vi "PDP Get Message.vi"(0 "Timeout ms (-1)":i32=-1) -> (1 "PDP Message Type":T1(ring), 2 "Text":string)   [LabVIEW 2009]
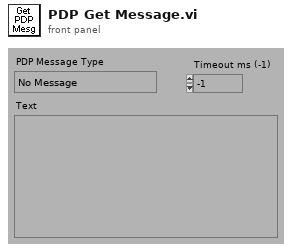
[diagram p1: front panel]
types:
  T1 = enum16{"No Message", "Bad Message", "RFFreq=", "RFMod=", "RFPower=", "QMeterName=", "YaleGain=", "ScanSweeps=", "ScanSteps=", "ScanFreq=", "Material=", "Baseline=", "CalConst=", "MonitorDelay=", "Channel=", "Channels=", "QCAPause", "QCATakeData", "QCANMRTune", "QCAMonitor", "Timer=", "LeadCurrent=", "LeadVoltage=", "MagCurrent=", "MagField=", "MagStatus=", "Setpoint=", "Setrate=", "HeaterDelay=", "Heater=", "HeaterDialog", "MagRemote", "MagLocal", "SendHe4Range", "uWaveFreq=", "uWavePower=", "BellowsPos=", "Event=", "Beep", "Message=", "Warning=", "Error=", "Address=", "Stop"}
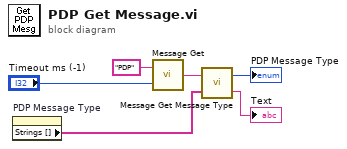
[diagram p0: block diagram]
diagram:
  n1 = property on="PDP Message Type" class="Enum (strict)"() -> ("Strings []"=w3:string[])  [unwired: 2 in, 2 out]
  n2 = call "Message Get.vi"("Timeout ms (-1)"="Timeout ms (-1)", "Module"="PDP") -> ("data out"=w6:string)
  n3 = call "Message Get Message Type.vi"("Message Types"=w3, "Message"=w6) -> ("Trailing text"=→"Text":string, "Message Type"=→"PDP Message Type":i32)
